vi "initialise_define_fp.vi"(8 "error in (no error)":errorcluster, 11 "TrajectoryMH100122AODRAPS in":refnum<class "TrajectoryMH100122AODRAPS.lvclass">) -> (0 "error out":errorcluster, 3 "TrajectoryMH100122AODRAPS out":refnum<class "TrajectoryMH100122AODRAPS.lvclass">)   [LabVIEW 2010, in "TrajectoryMH100122AODRAPS.lvclass"]
uses:
  TrajectoryMH100122AODRAPS.lvclass
  TrajectoryMH100122AODRAPS.lvclass/TrajectoryMH100122AODRAPS.ctl
  common/xcontrols/XImage/XImage/XImage.xctl
  class_data.vi
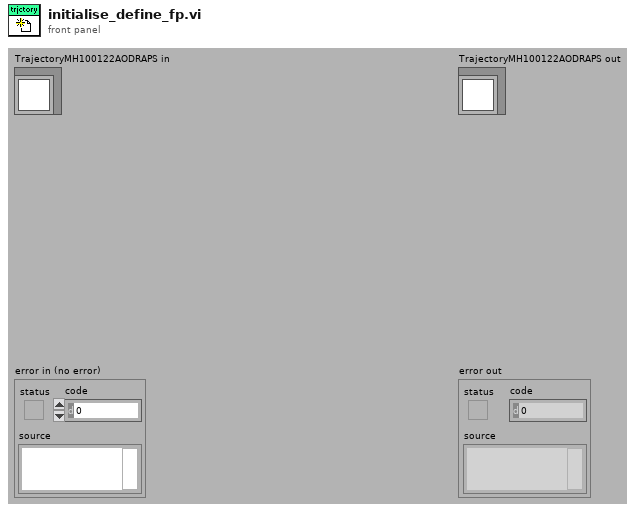
[diagram p1: front panel]
types:
  T1 = cluster{"Zoom Tool":bool, "Selection Tool":bool, "Pan Tool":bool, "Point Tool":bool, "Line Tool":bool, "Rectangle Tool":bool, "Rotated Rectangle Tool":bool, "Polyline Tool":bool, "Polygon Tool":bool, "Freehand Tool":bool, "Closed Freehand Tool":bool, "Ellipse Tool":bool, "Annulus Tool":bool}
  T2 = enum8{"Enabled", "Disabled", "Disabled and Grayed Out"}
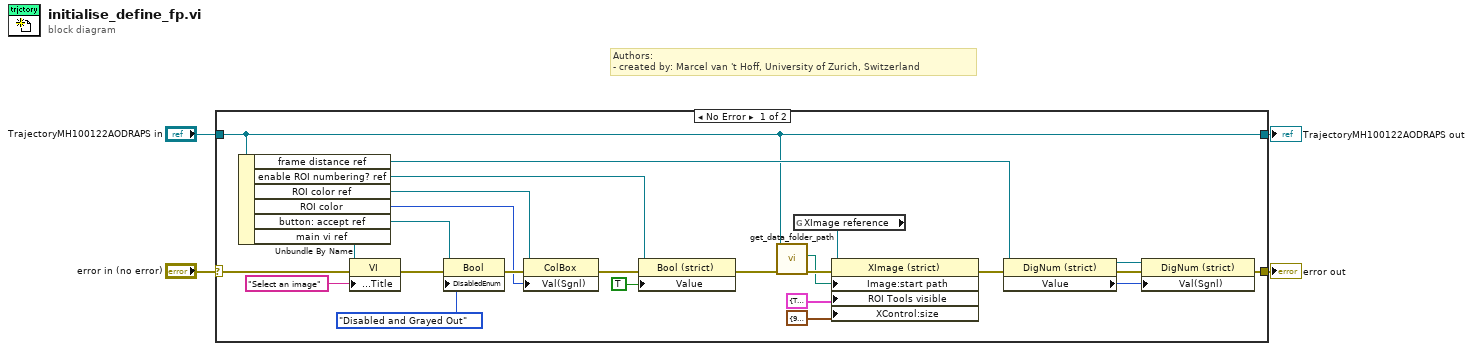
[diagram p0: block diagram]
diagram:
  # "Authors: \n- created by: Marcel van 't Hoff, University of Zurich, Switzerland"
  n1 = case shown="No Error" "error in (no error)" {
    selector: "error in (no error)" -> [w25 w31]
    tunnel: [w8 w31] -> w3
    tunnel: [w5 w30] -> w1
    tunnel: "TrajectoryMH100122AODRAPS in" -> [w5 w30]
    frame No Error {
      n2 = Unbundle By Name(w5) -> ("frame distance ref"=w14:refnum<vi>, "enable ROI numbering? ref"=w22:refnum<vi>, "ROI color ref"=w16:refnum<vi>, "ROI color"=w6:u32, "button: accept ref"=w28:refnum<vi>, "main vi ref"=w26:refnum<vi>)
      n3 = property class="VI"(reference=w26, error in=w25, "Front Panel.Title"="Select an image" ("Front Panel Window:Title")) -> (error out=w24:errorcluster)  [unwired: 1 out]
      n4 = property class="Bool"(reference=w28, error in=w24, "DisabledEnum"=T2."Disabled and Grayed Out" ("Disabled")) -> (error out=w23:errorcluster)  [unwired: 1 out]
      n5 = property class="ColBox"(reference=w16, error in=w23, "Val(Sgnl)"=w6) -> (error out=w7:errorcluster)  [unwired: 1 out]
      n6 = property class="Bool (strict)"(reference=w22, error in=w7, "Value"=TRUE) -> (error out=w19:errorcluster)  [unwired: 1 out]
      n7 = call-dynamic "get_data_folder_path.vi"("error in (no error)"=w19, "GenericComponent in"=w5) -> ("error out"=w18:errorcluster, "data folder path"=w17:path)  [unwired: 7 in, 1 out]
      n8 = global read "class_data.vi" "XImage reference"() -> (w20:refnum<vi>)
      n9 = property class="XImage (strict)"(reference=w20, error in=w18, "Image:start path"=w17, "ROI Tools visible"=T1 {"Zoom Tool"=TRUE, "Selection Tool"=TRUE, "Pan Tool"=TRUE, "Point Tool"=TRUE, "Line Tool"=TRUE, "Rectangle Tool"=FALSE, "Rotated Rectangle Tool"=FALSE, "Polyline Tool"=TRUE, "Polygon Tool"=FALSE, "Freehand Tool"=TRUE, "Closed Freehand Tool"=FALSE, "Ellipse Tool"=FALSE, "Annulus Tool"=FALSE} ("ROI:ROI Tools Palette visible"), "XControl:size"=cluster{"Width":u32, "Height":u32} {"Width"=915, "Height"=900}) -> (error out=w10:errorcluster)  [unwired: 1 out]
      n10 = property class="DigNum (strict)"(reference=w14, error in=w10) -> (reference out=w12:refnum<vi>, error out=w11:errorcluster, "Value"=w13:u16)
      n11 = property class="DigNum (strict)"(reference=w12, error in=w11, "Val(Sgnl)"=w13) -> (error out=w8:errorcluster)  [unwired: 1 out]
    }
    frame Error {
    }
  }
  "error out" <- w3
  "TrajectoryMH100122AODRAPS out" <- w1
